vi "test Parse File Info_2.vi"(11 "Test Case In":refnum<class "test Electronic Datasheet.lvclass">) -> (0 "error out":errorcluster, 3 "Test Case Out":refnum<class "test Electronic Datasheet.lvclass">)   [LabVIEW 2024, in "test Electronic Datasheet.lvclass"]
uses:
  test Electronic Datasheet.lvclass
  C:/Program Files/National Instruments/LabVIEW 2024/vi.lib/Astemes/LUnit/Test Case.lvclass
  <vilib>/PNR/JSONtext Object Serialization/Generic Object Serializer/Generic Object Serializer.lvclass
  C:/Program Files/National Instruments/LabVIEW 2024/vi.lib/JDP Science/JSONtext/LVClass Serializer/JSONtext LVClass Serializer.lvclass
  <vilib>/PNR/JSONtext Object Serialization/Generic Object Serializer/Type Name Handling.ctl
  <vilib>/PNR/JSONtext Object Serialization/Generic Object Serializer/Generic Object Serializer.lvclass/Generic Object Serializer.ctl
  <vilib>/Astemes/LUnit/Test Case.lvclass/Test Case.ctl
  99df47cb-525e-4171-a825-741cf93afc66.vi
  4993e8ee-a06a-463a-9684-69129f64d5ce.vi
  <vilib>/PNR/JSONtext Object Serialization/Generic Object Serializer/Write Type Name Handling.vi
  <vilib>/Astemes/LUnit/Append Pass Result.vi
  <vilib>/Astemes/LUnit/Append Fail Result.vi
  <vilib>/Astemes/LUnit/Describe Comparison.vi
  4993e8ee-a06a-463a-9684-69129f64d5ce.vi/9c5d11cd-9439-4240-a1ee-d9baace9c924.vi
  <vilib>/Astemes/LUnit/Run In UI.vi
  <vilib>/Utility/error.llb/Clear Errors.vi
  Electronic Datasheet/utils/Electronic Datasheet_GetAttributes.vi
  <vilib>/JDP Science/JSONtext/Variant to JSON Text.vi
  <vilib>/Astemes/LUnit/Describe Variant.vi
  Electronic Datasheet/Electronic Datasheet.lvclass
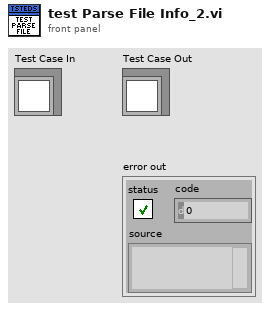
[diagram p1: front panel]
types:
  T1 = typedef "Generic Object Serializer.lvclass/Type Name Handling.ctl" = enum16{"None", "Inline"}
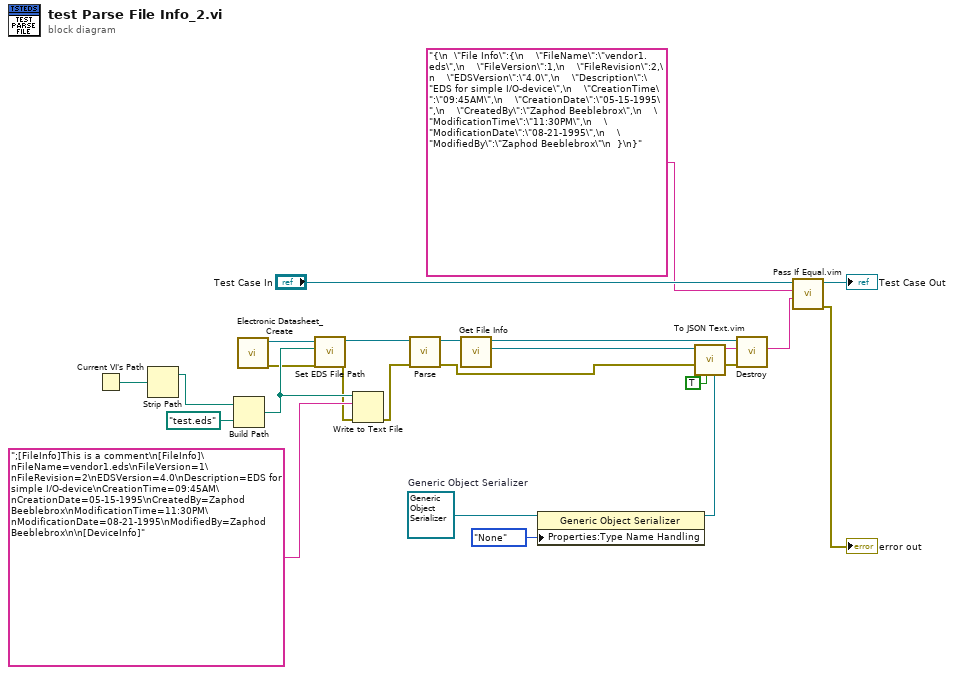
[diagram p0: block diagram]
diagram:
  w12 = refnum<class "Generic Object Serializer.lvclass"> refnum  # Generic Object Serializer
  n1 = Current VI's Path() -> (path=w20:path)
  n2 = Strip Path(path=w20) -> (stripped path=w19:path)  [unwired: 1 out]
  n3 = Build Path(base path=w19, name or relative path=path "test.eds") -> (appended path=w18:path)
  n4 = call "Electronic Datasheet_Create.vi"() -> ("Error Out"=w2:errorcluster, "reference out"=w3:refnum<class "Electronic Datasheet.lvclass">)  [unwired: 10 in]
  n5 = call "Set EDS File Path.vi"("error in"=w2, "EDS File Path"=w18, "reference in"=w3) -> ("error out"=w1:errorcluster, "reference out"=w21:refnum<class "Electronic Datasheet.lvclass">)  [unwired: 7 in]
  n6 = Write to Text File(file (use dialog)=w18, text=";[FileInfo]This is a comment\n[FileInfo]\nFileName=vendor1.eds\nFileVersion=1\nFileRevision=2\nEDSVersion=4.0\nDescription=EDS for simple I/O-device\nCreationTime=09:45AM\nCreationDate=05-15-1995\nCreatedBy=Zaphod Beeblebrox\nModificationTime=11:30PM\nModificationDate=08-21-1995\nModifiedBy=Zaphod Beeblebrox\n\n[DeviceInfo]", error in=w1) -> (error out=w16:errorcluster)  [unwired: 1 in, 2 out]
  n7 = call "Parse.vi"("error in"=w16, "reference in"=w21) -> ("error out"=w9:errorcluster, "reference out"=w14:refnum<class "Electronic Datasheet.lvclass">)  [unwired: 8 in]
  n8 = call "Get File Info.vi"("reference in"=w14) -> ("File Info"=w8:refnum<class "File Info.lvclass">, "reference out"=w5:refnum<class "Electronic Datasheet.lvclass">)  [unwired: 9 in]
  n9 = property class="Generic Object Serializer"(reference=w12, "Properties:Type Name Handling"=Type_Name_Handling."None" ("Type Name Handling")) -> (reference out=w11:refnum<class "Generic Object Serializer.lvclass">)  [unwired: 1 in, 1 out]
  n10 = call "To JSON Text.vim"("LVClass Serializer"=w11, "Pretty Print?"=TRUE, "error in (no error)"=w9, "Anything"=w8) -> ("error out"=w4:errorcluster, "<JSON>"=w7:string)  [unwired: 6 in]
  n11 = call-dynamic "Destroy.vi"("Error In"=w4, "reference in"=w5) -> ()  [unwired: 8 in, 2 out]
  n12 = call "Pass If Equal.vim"("Actual"=w7, "Expected"="{\n  \"File Info\":{\n    \"FileName\":\"vendor1.eds\",\n    \"FileVersion\":1,\n    \"FileRevision\":2,\n    \"EDSVersion\":\"4.0\",\n    \"Description\":\"EDS for simple I/O-device\",\n    \"CreationTime\":\"09:45AM\",\n    \"CreationDate\":\"05-15-1995\",\n    \"CreatedBy\":\"Zaphod Beeblebrox\",\n    \"ModificationTime\":\"11:30PM\",\n    \"ModificationDate\":\"08-21-1995\",\n    \"ModifiedBy\":\"Zaphod Beeblebrox\"\n  }\n}" ("<JSON>"), "LUnit Test Case In"="Test Case In") -> ("error out"=→"error out":errorcluster, "LUnit Test Case Out"=→"Test Case Out":refnum<class "test Electronic Datasheet.lvclass">)  [unwired: 7 in]
